vi "NMEA_经纬度转换.vi"(9 "类型":enum16{"Latitude", "Longitude"}(ring), 10 "数值":dbl) -> (2 "转换结果":string)   [LabVIEW 2016, in "环境动力监测库.lvlib" / "NMEA.lvlib"]
uses:
  NMEA.lvlib
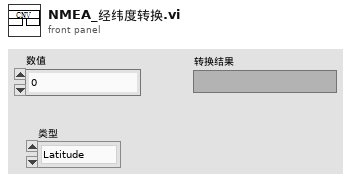
[diagram p1: front panel]
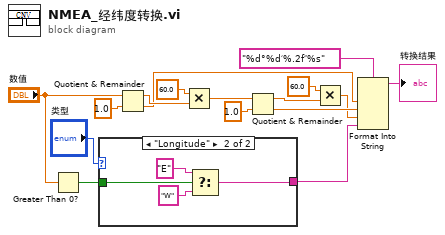
[diagram p0: block diagram]
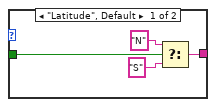
[diagram p2: hidden frame]
diagram:
  n1 = Greater Than 0?(x="数值") -> (x > 0?=w2:bool)
  n2 = case shown="\"Longitude\"" "类型" {
    tunnel: w2 -> [w20 w24]
    tunnel: [w17 w21] -> w1
    frame "Latitude", Default {
      n3 = Select(t="N" ("format string"), s=w20, f="S" ("format string")) -> (s? t:f=w17:string)
    }
    frame "Longitude" {
      n4 = Select(t="E" ("format string"), s=w24, f="W" ("format string")) -> (s? t:f=w21:string)
    }
  }
  n5 = Quotient & Remainder(x="数值", y=1.0) -> (x-y*floor(x/y)=w15:dbl, floor(x/y)=w8:dbl)
  n6 = Multiply(x=60.0, y=w15) -> (x*y=w13:dbl)
  n7 = Quotient & Remainder(x=w13, y=1.0) -> (x-y*floor(x/y)=w11:dbl, floor(x/y)=w7:dbl)
  n8 = Multiply(x=60.0, y=w11) -> (x*y=w6:dbl)
  n9 = Format Into String(format string="%d°%d′%.2f″%s", w8, w7, w6, w1) -> (resulting string=→"转换结果":string)  [unwired: 2 in, 1 out]
